vi "Write Local Msg Set.vi"(10 "Local Msg Set":T1, 11 "TEMPLATE Actor in":refnum<class "TEMPLATE Actor.lvclass">) -> (3 "TEMPLATE Actor out":refnum<class "TEMPLATE Actor.lvclass">)   [LabVIEW 2025, in "_Template.lvlib" / "Templates.lvlib" / "TEMPLATE Actor.lvlib" / "TEMPLATE Actor.lvclass"]
uses:
  TEMPLATE Actor.lvclass
  jettl/jettl/Msg Set.ctl
  jettl/jettl/Msg/Msg.lvclass
  TEMPLATE Actor.lvclass/TEMPLATE Actor.ctl
  jettl/jettl/jettl.lvlib
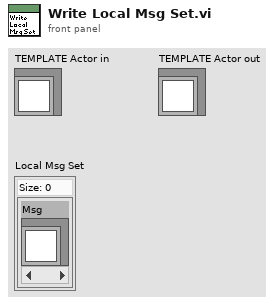
[diagram p1: front panel]
types:
  T1 = typedef "jettl.lvlib/Msg Set.ctl" = set{refnum<class "Msg.lvclass">}
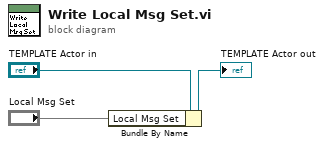
[diagram p0: block diagram]
diagram:
  n1 = Bundle By Name(cluster="TEMPLATE Actor in", "Local Msg Set"="Local Msg Set") -> (→"TEMPLATE Actor out":refnum<class "TEMPLATE Actor.lvclass">)
